vi "PRIME Detector Parse Time String.vi"(8 "error in":errorcluster, 11 "time string":string) -> (0 "error out":errorcluster, 3 "time":timestamp)   [LabVIEW 2021, in "PRIME Detector.lvclass"]
uses:
  PRIME Detector.lvclass
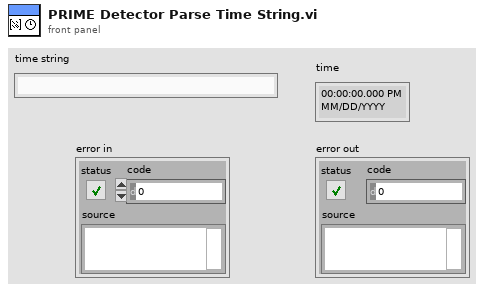
[diagram p1: front panel]
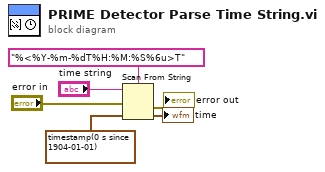
[diagram p0: block diagram]
diagram:
  n1 = Scan From String(format string="%<%Y-%m-%dT%H:%M:%S%6u>T", input string="time string", error in="error in", default 1=timestamp(0 s since 1904-01-01)) -> (error out=→"error out":errorcluster, output 1=→"time":timestamp)  [unwired: 1 in, 2 out]
